vi "Freeze_Threshold.vi"(0 "Path":path, 1 "Range":cluster{"Lower value":sgl, "Upper value":sgl}={"Lower value"=128.0, "Upper value"=255.0} {"Upper value" format="%.2f"; "Lower value" format="%.2f"}, 5 "Array":T1[](array[typedef]), 7 "RGB/Binary":enum32{"RGB", "Binary"}(radio), 9 "Image":i32, 11 "error in (no error)":errorcluster) -> (4 "Image out":T1, 6 "Numeric":i32, 15 "error out":errorcluster)   [LabVIEW 2022 SP3]
uses:
  <vilib>/vision/Image Controls.llb/IMAQ Image.ctl
  <vilib>/vision/NI_Vision_Development_Module.lvlib
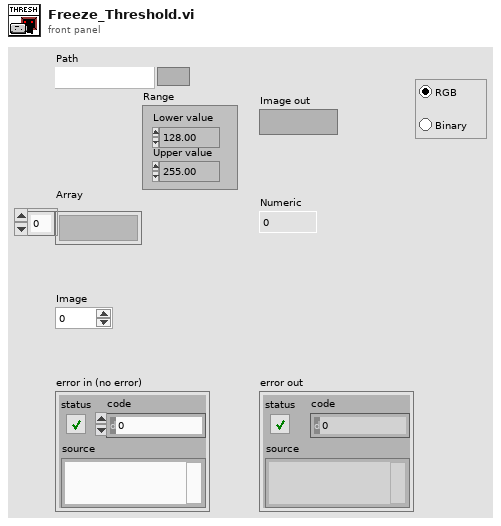
[diagram p1: front panel]
types:
  T1 = typedef "IMAQ Image.ctl" = refnum<image>
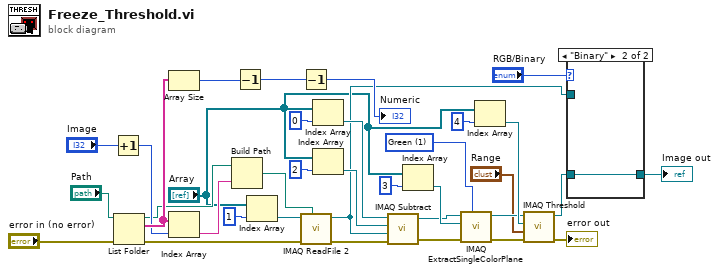
[diagram p0: block diagram]
diagram:
  w6 = 1 items=["Red", "Green", "Blue", "Hue", "Saturation", "Luminance", "Value", "Intensity"] ("Color Plane")
  n1 = Increment(x="Image") -> (x+1=w21:i32)
  n2 = List Folder(path="Path", error in="error in (no error)") -> (path out=w18:path, filenames=w29:string[], error out=w19:errorcluster)  [unwired: 2 in, 1 out]
  n3 = Array Size(array=w29) -> (size(s)=w30:i32)
  n4 = Index Array(array=w29, index=w21) -> (element=w23:string)
  n5 = Build Path(base path=w18, name or relative path=w23) -> (appended path=w22:path)
  n6 = Decrement(x=w30) -> (x-1=w28:i32)
  n7 = Index Array(array="Array", index=1) -> (element=w25:T1)
  n8 = Decrement(x=w28) -> (x-1=→"Numeric":i32)
  n9 = call "IMAQ ReadFile 2"("File Path"=w22, "error in (no error)"=w19, "Image"=w25) -> ("error out"=w35:errorcluster, "Image Out"=w14:T1)  [unwired: 4 in, 3 out]
  n10 = Index Array(array="Array", index=0) -> (element=w34:T1)
  n11 = Index Array(array="Array", index=2) -> (element=w32:T1)
  n12 = call "IMAQ Subtract"("Image Src A"=w34, "Image Dst"=w32, "Image Src B"=w14, "error in (no error)"=w35) -> ("Image Dst Out"=w7:T1, "error out"=w1:errorcluster)  [unwired: 3 in]
  n13 = Index Array(array="Array", index=3) -> (element=w8:T1)
  n14 = call "IMAQ ExtractSingleColorPlane"("Color Plane"=w6, "error in (no error)"=w1, "Image Dst"=w8, "Image Src"=w7) -> ("error out"=w11:errorcluster, "Image Dst Out"=w5:T1)  [unwired: 6 in]
  n15 = Index Array(array="Array", index=4) -> (element=w12:T1)
  n16 = call "IMAQ Threshold"("error in (no error)"=w11, "Range"="Range", "Image Dst"=w12, "Image Src"=w5) -> ("error out"=→"error out":errorcluster, "Image Dst Out"=w4:T1)  [unwired: 6 in]
  n17 = case shown="\"Binary\"" "RGB/Binary" {
    tunnel: w4 -> [_ w37]
    tunnel: [w36 w37] -> w16
    tunnel: w14 -> [w36 _]
    frame "RGB", Default {
    }
    frame "Binary" {
    }
  }
  "Image out" <- w16
